vi "释放.vi"(8 "error in (no error)":errorcluster caption="错误输入（无错误）", 11 "堆栈(DBL) 输入":refnum<class "堆栈(U16).lvclass"> caption="DNL_LabVIEW Object in") -> (0 "error out":errorcluster caption="错误输出")   [LabVIEW 2011, in "堆栈(U16).lvclass"]
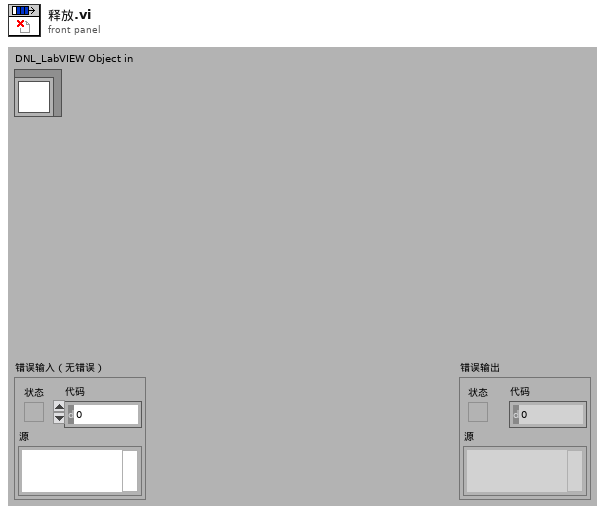
[diagram p1: front panel]
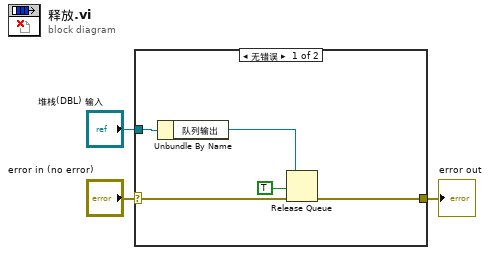
[diagram p0: block diagram]
diagram:
  n1 = case shown="无错误" "error in (no error)" {
    selector: "error in (no error)" -> [w7 w9]
    tunnel: [w6 w9] -> w2
    tunnel: "堆栈(DBL) 输入" -> [w8 _]
    frame No Error {
      n2 = Unbundle By Name(w8) -> ("队列输出"=w4:refnum<queue>)
      n3 = Release Queue(queue=w4, force destroy? (F)=TRUE ("强制销毁？(F)"), error in (no error)=w7) -> (error out=w6:errorcluster)  [unwired: 2 out]
    }
    frame Error {
    }
  }
  "error out" <- w2
